vi "Error Handler.vi"(8 "error in (no error)":errorcluster, 11 "Status":i32) -> (0 "error out":errorcluster)   [LabVIEW 2013, in "Vaunix LDA.lvlib"]
doc: "Decodes and errors that the functions in the API may generate. The error codes and what they represent are outlined in the 'VNX_LDA_api.h' header file."
uses:
  Attenuator_Vaunix-LDA_LabView_32Bit_Driver/Vaunix LDA/Vaunix LDA.lvlib
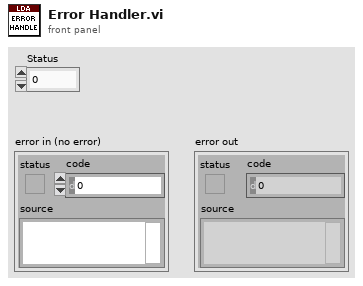
[diagram p1: front panel]
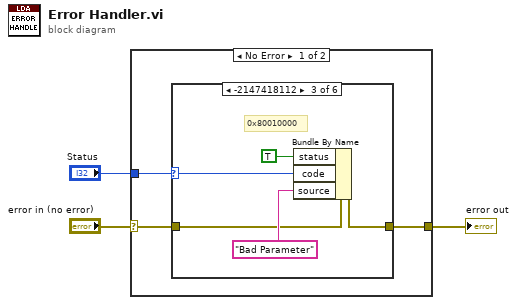
[diagram p0: block diagram]
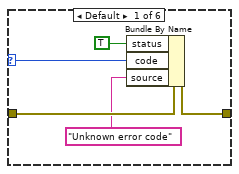
[diagram p2: hidden frame]
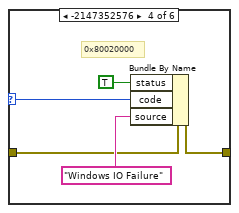
[diagram p4: hidden frame]
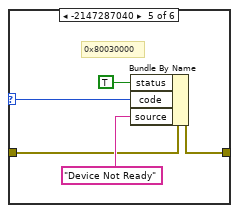
[diagram p5: hidden frame]
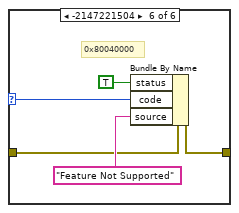
[diagram p6: hidden frame]
diagram:
  n1 = case shown="No Error" "error in (no error)" {
    selector: "error in (no error)" -> [w4 w33]
    tunnel: [w5 w33] -> w2
    tunnel: "Status" -> [w6 _]
    frame No Error {
      n2 = case shown="-2147418112" w6 {
        selector: w6 -> [w9 _ w15 w20 w25 w30]
        tunnel: [w10 w12 w13 w18 w23 w28] -> w5
        tunnel: w4 -> [w11 w12 w14 w19 w24 w29]
        frame Default {
          n3 = Bundle By Name(cluster=w11, "status"=TRUE, "code"=w9, "source"="Unknown error code") -> (w10:errorcluster)
        }
        frame 0 {
          # "No Error"
        }
        frame -2147418112 {
          # "0x80010000"
          n4 = Bundle By Name(cluster=w14, "status"=TRUE, "code"=w15, "source"="Bad Parameter") -> (w13:errorcluster)
        }
        frame -2147352576 {
          # "0x80020000"
          n5 = Bundle By Name(cluster=w19, "status"=TRUE, "code"=w20, "source"="Windows IO Failure") -> (w18:errorcluster)
        }
        frame -2147287040 {
          # "0x80030000"
          n6 = Bundle By Name(cluster=w24, "status"=TRUE, "code"=w25, "source"="Device Not Ready") -> (w23:errorcluster)
        }
        frame -2147221504 {
          # "0x80040000"
          n7 = Bundle By Name(cluster=w29, "status"=TRUE, "code"=w30, "source"="Feature Not Supported") -> (w28:errorcluster)
        }
      }
    }
    frame Error {
      # "There was a LabView error or an existing error.\nPass it through unaltered."
    }
  }
  "error out" <- w2
